vi "Controller.vi"(8 "error in (no error)":errorcluster, 10 "Tanks levels":dbl[](array[numeric])) -> (0 "error out":errorcluster, 2 "Pumps Voltages":dbl[](array[numeric]), 5 "Plant Control Variables":T1)   [LabVIEW 2018]
uses:
  <vilib>/Simulation/Shared/_Datatypes/SIM MIMO State Space.ctl
  <vilib>/Simulation/DiscreteLinear/Implementation/NILVSim Discrete State Space Direct.llb/SIM Discrete State Space Direct Diagram (MIMO).vi
  <vilib>/Simulation/DiscreteLinear/Implementation/Shared/SIM Init Discrete States.vi
  <vilib>/Simulation/DiscreteLinear/Implementation/NILVSim Discrete State Space Direct.llb/NILVSim Discrete State Space Direct Diagram Core (MIMO).vi
  <vilib>/Simulation/Implementation/Shared/SIM BuildSimErr.vi
  <vilib>/Simulation/Implementation/XNodeFramework/SimXNode/SimX.xnode
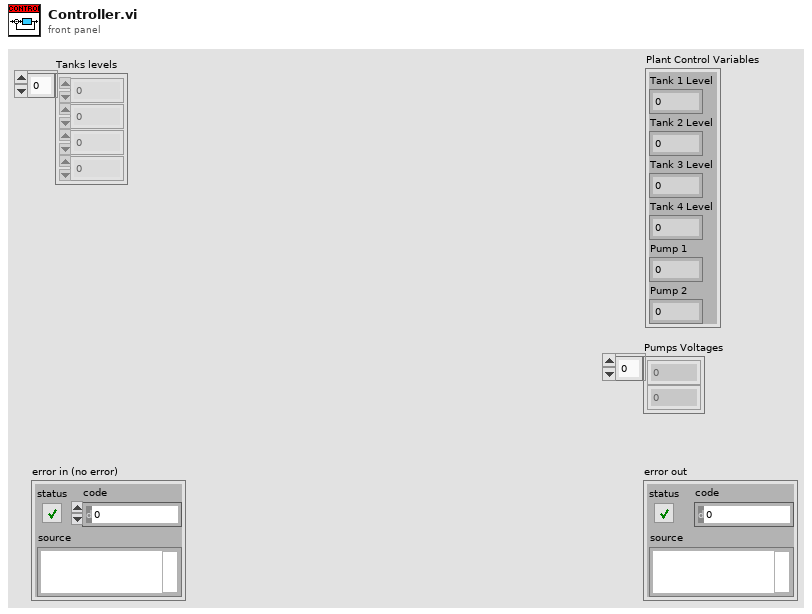
[diagram p1: front panel]
types:
  T1 = cluster{"Tank 1 Level":dbl, "Tank 2 Level":dbl, "Tank 3 Level":dbl, "Tank 4 Level":dbl, "Pump 1":dbl, "Pump 2":dbl}
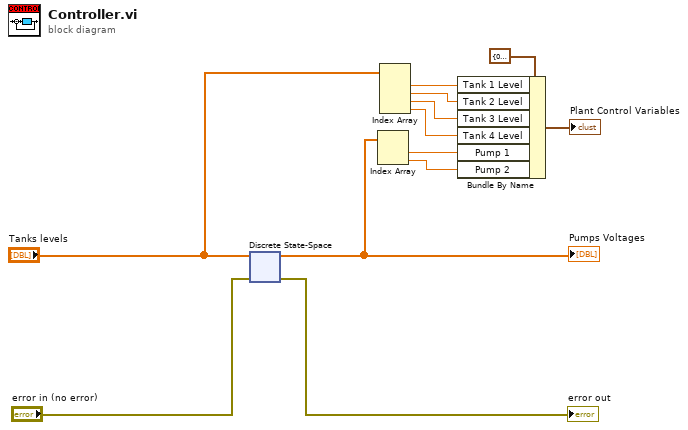
[diagram p0: block diagram]
diagram:
  n1 = xnode "Discrete State-Space"("input u(k)"="Tanks levels", "error in (no error)"="error in (no error)") -> ("output y(k)"=w8:dbl[], "error out"=→"error out":errorcluster)  [unwired: 1 in, 2 out]
  "Pumps Voltages" <- w8
  n2 = Index Array(array=w8) -> (element #1=w7:dbl, element #2=w6:dbl)  [unwired: 2 in]
  n3 = Index Array(array="Tanks levels") -> (element #1=w5:dbl, element #2=w3:dbl, element #3=w2:dbl, element #4=w1:dbl)  [unwired: 4 in]
  n4 = Bundle By Name(cluster=T1 {"Tank 1 Level"=0.0, "Tank 2 Level"=0.0, "Tank 3 Level"=0.0, "Tank 4 Level"=0.0, "Pump 1"=0.0, "Pump 2"=0.0} ("Plant Control Variables"), "Tank 1 Level"=w5, "Tank 2 Level"=w3, "Tank 3 Level"=w2, "Tank 4 Level"=w1, "Pump 1"=w7, "Pump 2"=w6) -> (→"Plant Control Variables":T1)
